vi "variant2Attributes.vi"(0 "HGF_DIMSubscriber":refnum<class "HGF_DIMSubscriber.lvclass">, 2 "rawData":variant, 3 "typeDescriptor":string, 5 "error in (no error)":errorcluster) -> (14 "HGF_DIMSubscriber":refnum<class "HGF_DIMSubscriber.lvclass">, 15 "no link":bool, 16 "Parameter":variant, 17 "typeDescriptor":string, 19 "error out":errorcluster)   [LabVIEW 2012, in "HGF_DIM.lvlib" / "HGF_DIMSubscriber.lvclass"]
doc: "Convert raw data value of variant to variant attributes Pn, n=0,1,2,..."
uses:
  HGF_DIMSubscriber.lvclass
  HGF_BaseClasses/HGF_PVSubscriber/HGF_PVSubscriber.lvclass
  DimLVEvent/LVDimInterface/LVDimInterface.lvlib
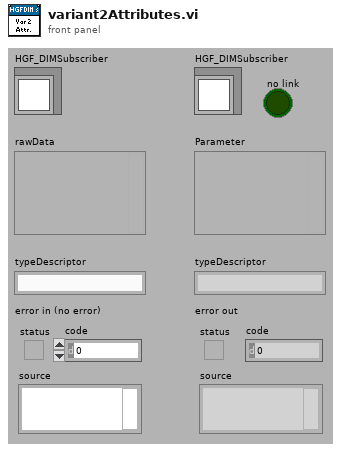
[diagram p1: front panel]
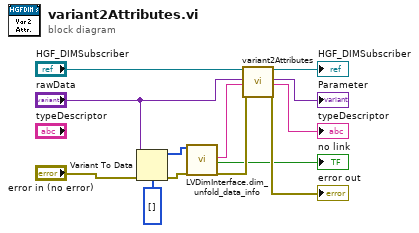
[diagram p0: block diagram]
diagram:
  n1 = Variant To Data(error in="error in (no error)", type=i8[] [], Variant="rawData") -> (data=w5:i8[], error out=w4:errorcluster)
  n2 = call "LVDimInterface.dim_unfold_data_info.vi"("rawData"=w5, "error in (no error)"=w4) -> ("typeDescriptor"=w2:string, "no link"=→"no link":bool, "error out"=w3:errorcluster)  [unwired: 15 out]
  n3 = call-parent "variant2Attributes.vi"("HGV_PVBase"="HGF_DIMSubscriber", "rawData"="rawData", "typeDescriptor"=w2, "error in (no error)"=w3) -> ("HGV_PVBase"=→"HGF_DIMSubscriber":refnum<class "HGF_DIMSubscriber.lvclass">, "Parameter"=→"Parameter":variant, "typeDescriptor"=→"typeDescriptor":string, "error out"=→"error out":errorcluster)  [unwired: 12 out]
